vi "Set Alarm to 12 o Clock.vi"(0 "Limits":cluster{"Low Limit":dbl, "Hi Limit":dbl}, 1 "Knob Refnum":refnum<vi>) -> ()   [LabVIEW 2018]
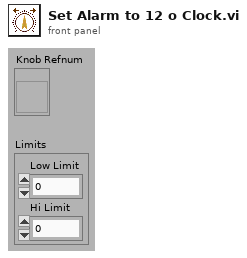
[diagram p1: front panel]
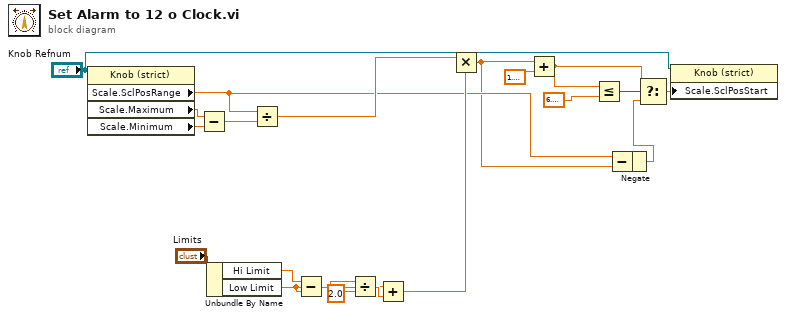
[diagram p0: block diagram]
diagram:
  n1 = property on="Property Node" class="Knob (strict)"(reference="Knob Refnum") -> ("Scale.SclPosRange"=w5:dbl, "Scale.Maximum"=w7:dbl, "Scale.Minimum"=w11:dbl)  [unwired: 1 in, 2 out]
  n2 = Subtract(x=w7, y=w11) -> (x-y=w12:dbl)
  n3 = Unbundle By Name("Limits") -> ("Hi Limit"=w16:dbl, "Low Limit"=w20:dbl)
  n4 = Divide(x=w5, y=w12) -> (x/y=w8:dbl)
  n5 = Subtract(x=w16, y=w20) -> (x-y=w17:dbl)
  n6 = Divide(x=w17, y=2.0) -> (x/y=w19:dbl)
  n7 = Add(x=w19, y=w20) -> (x+y=w21:dbl)
  n8 = Multiply(x=w8, y=w21) -> (x*y=w4:dbl)
  n9 = Add(x=w4, y=1.5707963267948966) -> (x+y=w6:dbl)
  n10 = Less Or Equal?(x=w6, y=6.283185307179586) -> (x <= y?=w13:bool)
  n11 = Subtract(x=w5, y=w4) -> (x-y=w3:dbl)
  n12 = Negate(x=w3) -> (-x=w2:dbl)
  n13 = Select(t=w6, s=w13, f=w2) -> (s? t:f=w14:dbl)
  n14 = property on="Property Node" class="Knob (strict)"(reference="Knob Refnum", "Scale.SclPosStart"=w14) -> ()  [unwired: 1 in, 2 out]
